vi "TRIODE Experiment.vi"() -> ()   [LabVIEW 2020]
uses:
  Typedef_SerialFGVActions.ctl
  <vilib>/Utility/file.llb/Write To Spreadsheet File (DBL).vi
panel:
  in  "No. of steps in Scan loop":i32=4096
  in  "Tab Control":enum32{"ANODE Scan", "GRID Scan"}(tab)
  out "Total ANODE scan":cluster{dbl[], dbl[]}[](graph)
  in  "Start Anode Scan":bool
  in  "-ve GRID Increment Voltage (V)":dbl
  in  "-ve GRID End Voltage (V)":dbl
  in  "-ve GRID Start Voltage (V)":dbl
  out "Individual ANODE scan":cluster{dbl[], dbl[]}(graph)
  in  "Start GRID scan":bool
  in  "+ve ANODE Start Voltage (V)":dbl
  in  "+ve ANODE End Voltage (V)":dbl
  in  "ANODE Increment Voltage (V)":dbl
  out "Individual GRID Scan":cluster{dbl[], dbl[]}(graph)
  out "Total GRID Scan":cluster{dbl[], dbl[]}[](graph)
  out "Filament Current Monitor Graph":dbl[](graph)
  in  "VISA resource name":refnum<visa-resource-name>="COM10"
  # "NOTE this needs to be set \nto the correct COM port \nas used by the Control System"
  # "This sets how many data points\nare used for a single scan"
  # "DAC 0 is GRID voltage\n\nDAC 1 is ANODE voltage\n\nADC0 is Filament Current (should be constant)\n\nADC1 is Anode Current (to be measured)\n\nADC2 is GRID Voltage monitor\n\nADC3 is ANODE Voltage Monitor"
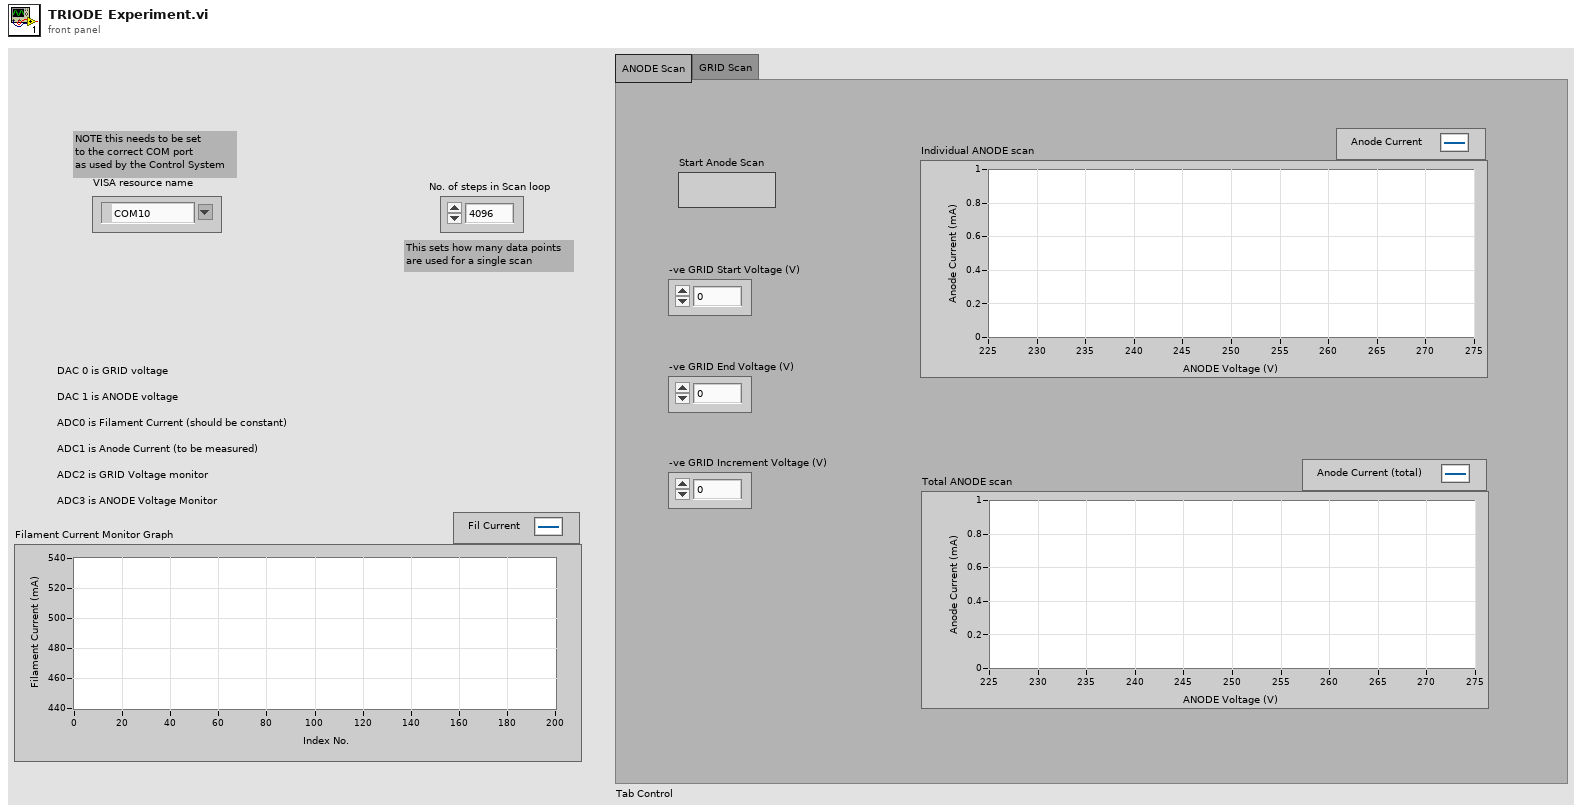
[diagram p1: front panel]
types:
  T1 = typedef "Typedef_SerialFGVActions.ctl" = enum16{"Open Serial Port", "Close Serial Port", "Update DAC", "Read ADC", "Read All ADCs"}
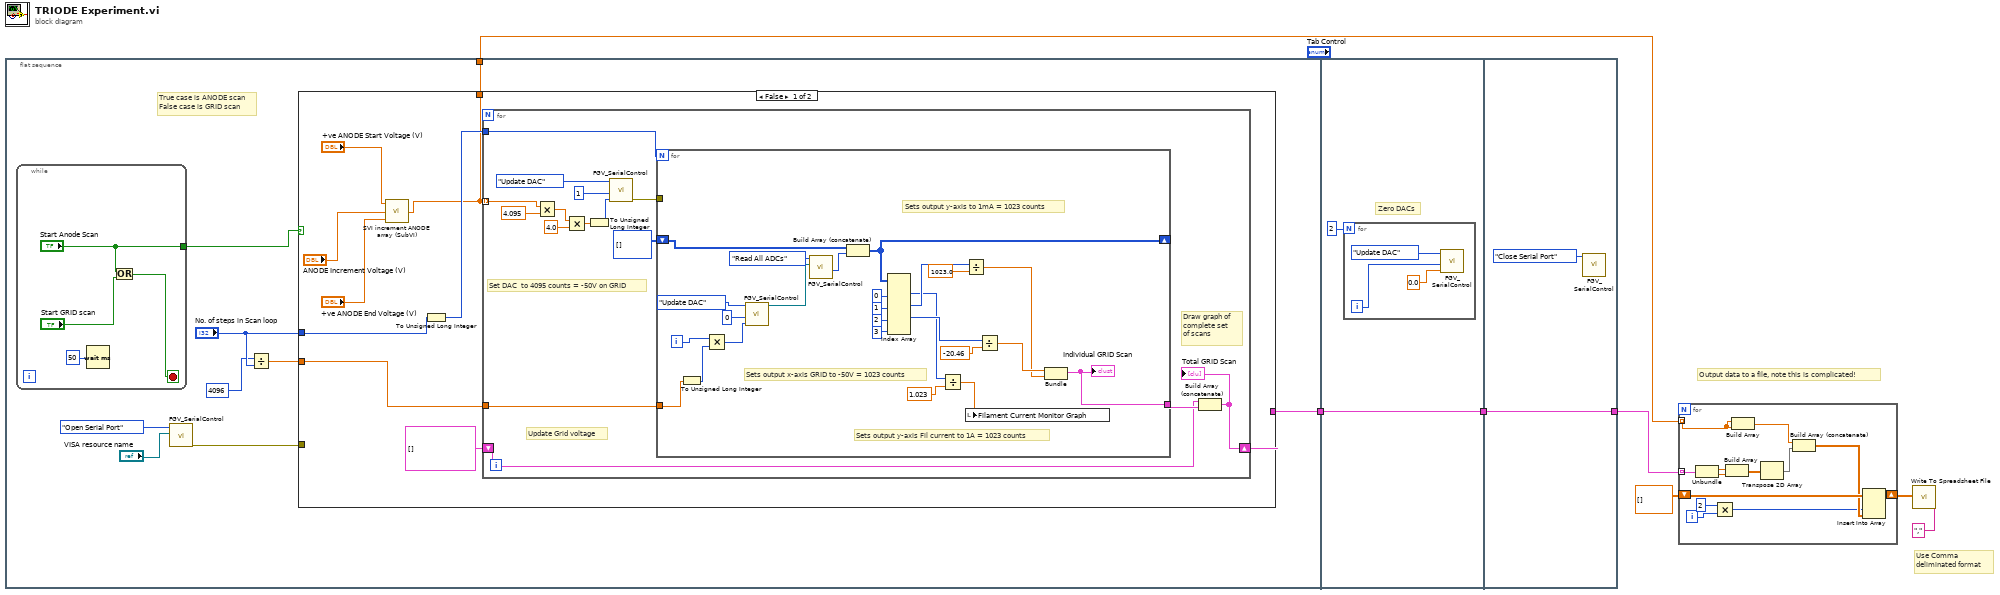
[diagram p0: block diagram]
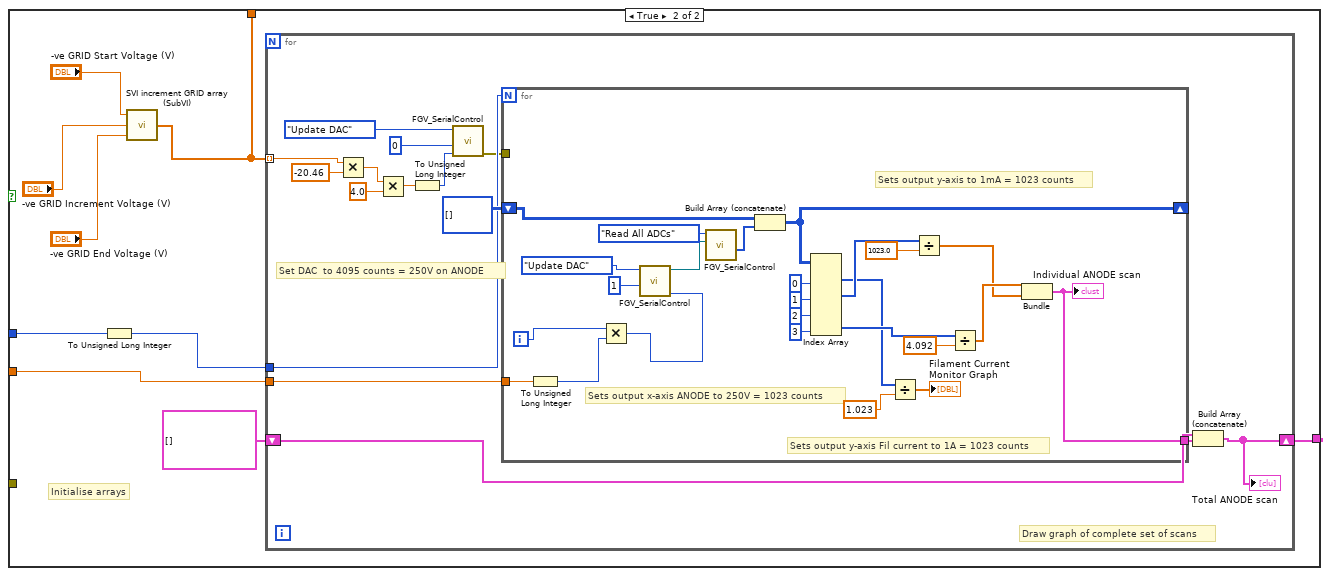
[diagram p2: hidden frame]
diagram:
  # "Use Comma \ndeliminated format"
  # "Output data to a file, note this is complicated!"
  n1 = flat-sequence {
    tunnel: [w9] -> w6
    tunnel: [w8] -> w5
    tunnel: [w119] -> w7
    tunnel: w6 -> [w119]
    tunnel: w7 -> [w124]
    tunnel: [w124] -> w4
    frame #0 {
      # "True case is ANODE scan\nFalse case is GRID scan"
      n2 = while {
        tunnel: ["Start Anode Scan"] -> w13
        stop <- w19 stop-if-true
        n3 = Wait (ms)(milliseconds to wait=u32 50) -> ()  [unwired: 1 out]
        n4 = Or(x="Start Anode Scan", y="Start GRID scan") -> (x .or. y?=w19:bool)
      }
      n5 = call "FGV_SerialControl.vi"("Action"=Typedef_SerialFGVActions."Open Serial Port", "VISA Refnum in"="VISA resource name") -> ("error out"=w14:errorcluster)  [unwired: 5 in, 3 out]
      n6 = Divide(x=4096, y="No. of steps in Scan loop") -> (x/y=w11:dbl)
      n7 = case shown="False" w13 {
        tunnel: w14 -> [_ _]
        tunnel: w11 -> [w25 w74]
        tunnel: "No. of steps in Scan loop" -> [w24 w73]
        tunnel: [w21 w71] -> w9
        tunnel: [w22 w70] -> w8
        frame False {
          n8 = call "SVI increment ANODE array (SubVI).vi"("End Voltage (V)"="+ve ANODE End Voltage (V)", "Increment Voltage (V)"="ANODE Increment Voltage (V)", "Start Voltage (V)"="+ve ANODE Start Voltage (V)") -> ("output"=w22:dbl[])
          n9 = To Unsigned Long Integer(number=w24) -> (unsigned 32bit integer=w26:u32)
          n10 = for {
            tunnel: w22 -> [w38] mode=indexing
            tunnel: w25 -> [w37]
            tunnel: w26 -> [w36]
            shift-right: [w30] -> w21
            shift-left: cluster{dbl[], dbl[]}[] [] -> [w31]
            # "Draw graph of \ncomplete set \nof scans"
            # "Set DAC  to 4095 counts = -50V on GRID"
            # "Update Grid voltage"
            n11 = Multiply(x=w38, y=4.095) -> (x*y=w41:dbl)
            n12 = Multiply(x=w41, y=4.0) -> (x*y=w35:dbl)
            n13 = To Unsigned Long Integer(number=w35) -> (unsigned 32bit integer=w34:u32)
            n14 = call "FGV_SerialControl.vi"("Action"=Typedef_SerialFGVActions."Update DAC", "Channel"=u8 1, "Voltage"=w34) -> ("error out"=w33:errorcluster)  [unwired: 4 in, 3 out]
            n15 = for {
              N: w36 -> [_]
              shift-right: [w53] -> _
              shift-left: u16[][] [] -> [w52]
              tunnel: w37 -> [w50]
              tunnel: w33 -> [_]
              tunnel: [w45] -> w32
              i -> [w48]
              # "Sets output y-axis Fil current to 1A = 1023 counts"
              # "Sets output x-axis GRID to -50V = 1023 counts"
              # "Sets output y-axis to 1mA = 1023 counts"
              n16 = To Unsigned Long Integer(number=w50) -> (unsigned 32bit integer=w47:u32)
              n17 = Multiply(x=w48, y=w47) -> (x*y=w49:u32)
              n18 = call "FGV_SerialControl.vi"("Action"=Typedef_SerialFGVActions."Update DAC", "Channel"=u8 0, "Voltage"=w49) -> ("VISA Refnum out"=w46:refnum<visa-resource-name>)  [unwired: 4 in, 3 out]
              n19 = call "FGV_SerialControl.vi"("Action"=Typedef_SerialFGVActions."Read All ADCs", "VISA Refnum in"=w46) -> ("Voltages"=w59:u16[])  [unwired: 5 in, 3 out]
              n20 = Build Array (concatenate)(w52, w59) -> (w53:u16[][])
              n21 = Index Array(array=w53, index (col) #1=0 ("disabled index (col)"), index (col) #2=1 ("index (col)"), index (col) #3=2 ("index (col)"), index (col) #4=3 ("index (col)")) -> (element #1=w61:u16[], element #2=w63:u16[], element #3=w66:u16[])  [unwired: 4 in, 1 out]
              n22 = Divide(x=w61, y=1.023) -> (x/y=w51:dbl[])
              n23 = Divide(x=w63, y=1023.0) -> (x/y=w64:dbl[])
              n24 = local write "Filament Current Monitor Graph"(w51) -> ()
              n25 = Divide(x=w66, y=-20.46) -> (x/y=w67:dbl[])
              n26 = Bundle(w67, w64) -> (w45:cluster{dbl[], dbl[]})  [unwired: 1 in]
              "Individual GRID Scan" <- w45
            }
            n27 = Build Array (concatenate)(w31, w32) -> (w30:cluster{dbl[], dbl[]}[])
            "Total GRID Scan" <- w30
          }
        }
        frame True {
          # "Initialise arrays"
          n28 = To Unsigned Long Integer(number=w73) -> (unsigned 32bit integer=w75:u32)
          n29 = call "SVI increment GRID array (SubVI).vi"("End Voltage (V)"="-ve GRID End Voltage (V)", "Increment Voltage (V)"="-ve GRID Increment Voltage (V)", "Start Voltage (V)"="-ve GRID Start Voltage (V)") -> ("output"=w70:dbl[])
          n30 = for {
            tunnel: w70 -> [w90] mode=indexing
            tunnel: w75 -> [w86]
            tunnel: w74 -> [w85]
            shift-right: [w79] -> w71
            shift-left: cluster{dbl[], dbl[]}[] [] -> [w80]
            # "Draw graph of complete set of scans"
            # "Set DAC  to 4095 counts = 250V on ANODE"
            n31 = Multiply(x=w90, y=-20.46) -> (x*y=w89:dbl)
            n32 = Multiply(x=w89, y=4.0) -> (x*y=w84:dbl)
            n33 = To Unsigned Long Integer(number=w84) -> (unsigned 32bit integer=w83:u32)
            n34 = call "FGV_SerialControl.vi"("Action"=Typedef_SerialFGVActions."Update DAC", "Channel"=u8 0, "Voltage"=w83) -> ("error out"=w82:errorcluster)  [unwired: 4 in, 3 out]
            n35 = for {
              N: w86 -> [_]
              shift-right: [w101] -> _
              shift-left: u16[][] [] -> [w100]
              tunnel: w85 -> [w99]
              tunnel: w82 -> [_]
              tunnel: [w94] -> w81
              i -> [w98]
              # "Sets output y-axis Fil current to 1A = 1023 counts"
              # "Sets output x-axis ANODE to 250V = 1023 counts"
              # "Sets output y-axis to 1mA = 1023 counts"
              n36 = To Unsigned Long Integer(number=w99) -> (unsigned 32bit integer=w97:u32)
              n37 = Multiply(x=w98, y=w97) -> (x*y=w96:u32)
              n38 = call "FGV_SerialControl.vi"("Action"=Typedef_SerialFGVActions."Update DAC", "Channel"=u8 1, "Voltage"=w96) -> ("VISA Refnum out"=w95:refnum<visa-resource-name>)  [unwired: 4 in, 3 out]
              n39 = call "FGV_SerialControl.vi"("Action"=Typedef_SerialFGVActions."Read All ADCs", "VISA Refnum in"=w95) -> ("Voltages"=w107:u16[])  [unwired: 5 in, 3 out]
              n40 = Build Array (concatenate)(w100, w107) -> (w101:u16[][])
              n41 = Index Array(array=w101, index (col) #1=0 ("disabled index (col)"), index (col) #2=1 ("index (col)"), index (col) #3=2 ("index (col)"), index (col) #4=3 ("index (col)")) -> (element #1=w109:u16[], element #2=w112:u16[], element #4=w115:u16[])  [unwired: 4 in, 1 out]
              n42 = Divide(x=w109, y=1.023) -> (x/y=→"Filament Current Monitor Graph":dbl[])
              n43 = Divide(x=w112, y=1023.0) -> (x/y=w113:dbl[])
              n44 = Divide(x=w115, y=4.092) -> (x/y=w116:dbl[])
              n45 = Bundle(w116, w113) -> (w94:cluster{dbl[], dbl[]})  [unwired: 1 in]
              "Individual ANODE scan" <- w94
            }
            n46 = Build Array (concatenate)(w80, w81) -> (w79:cluster{dbl[], dbl[]}[])
            "Total ANODE scan" <- w79
          }
        }
      }
    }
    frame #1 {
      # "Zero DACs"
      n47 = for {
        N: 2 -> [_]
        i -> [w122]
        n48 = call "FGV_SerialControl.vi"("Action"=Typedef_SerialFGVActions."Update DAC", "Channel"=w122, "Voltage"=0.0) -> ()  [unwired: 4 in, 4 out]
      }
    }
    frame #2 {
      n49 = call "FGV_SerialControl.vi"("Action"=Typedef_SerialFGVActions."Close Serial Port") -> ()  [unwired: 6 in, 4 out]
    }
  }
  n50 = for {
    tunnel: w4 -> [w138] mode=indexing
    tunnel: w5 -> [w135] mode=indexing
    shift-right: [w131] -> w2
    shift-left: dbl[][] [] -> [w130]
    i -> [w128]
    n51 = Unbundle(w138) -> (w136:dbl[], w137:dbl[])
    n52 = Multiply(x=2, y=w128) -> (x*y=w126:i32)
    n53 = Build Array(w136, w137) -> (w133:dbl[][])
    n54 = Build Array(w135, w135) -> (w134:dbl[])
    n55 = Transpose 2D Array(2D array=w133) -> (transposed array=w132:dbl[][])
    n56 = Build Array (concatenate)(w134, w132) -> (w129:dbl[][])
    n57 = Insert Into Array(array=w130, index (col)=w126, new element=w129) -> (w131:dbl[][])  [unwired: 1 in]
  }
  n58 = call-poly <vilib>:"Write To Spreadsheet File.vi"("delimiter (\\t)"="," ("delimiter (\\t)"), "2D data"=w2) -> ()  [unwired: 6 in, 1 out]
